vi "Read Done_.vi"(8 "error in (no error)":errorcluster, 11 "TCPReceiver in":refnum<class "TCPReceiver.lvclass">) -> (0 "error out":errorcluster, 2 "Done?":bool, 3 "TCPReceiver out":refnum<class "TCPReceiver.lvclass">)   [LabVIEW 2019, in "TCPReceiver.lvclass"]
uses:
  TCPReceiver.lvclass
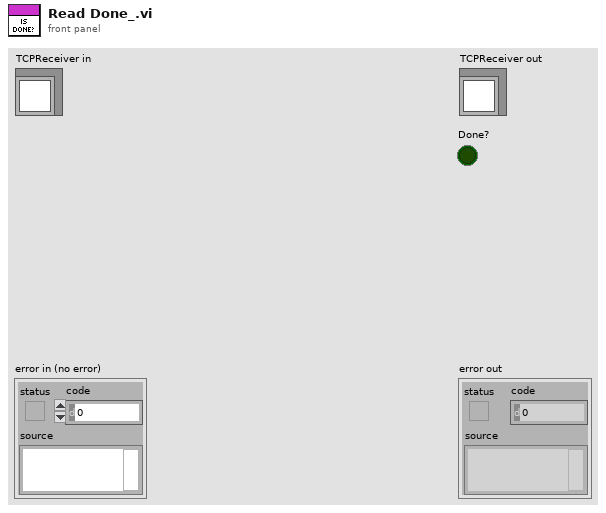
[diagram p1: front panel]
types:
  T1 = typedef "TCPReceiver.lvclass/TCPReceiver Progress STYP.ctl" = cluster{"HeaderSize?":bool, "Header?":bool, "Body?":bool}
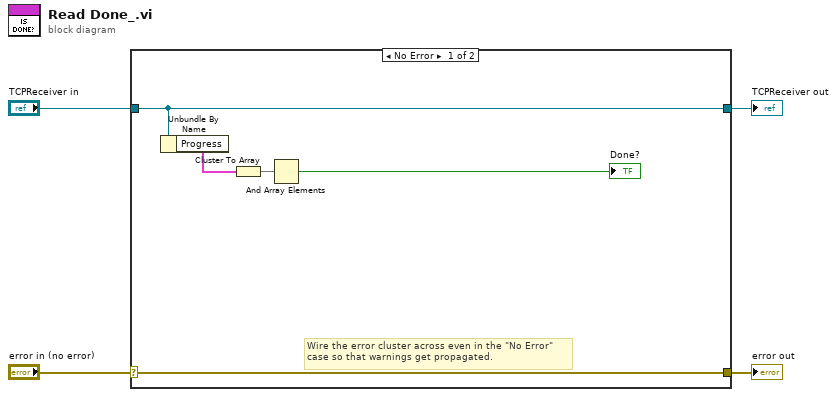
[diagram p0: block diagram]
diagram:
  n1 = case shown="No Error" "error in (no error)" {
    selector: "error in (no error)" -> [w9 w11]
    tunnel: [w9 w11] -> w3
    tunnel: [w8 w10] -> w1
    tunnel: "TCPReceiver in" -> [w8 w10]
    frame No Error {
      # "Wire the error cluster across even in the \"No Error\"\ncase so that warnings get propagated."
      n2 = Unbundle By Name(w8) -> ("Progress"=w7:T1)
      n3 = Cluster To Array(cluster=w7) -> (array=w6:bool[])
      n4 = And Array Elements(Boolean array=w6) -> (logical AND=→"Done?":bool)
    }
    frame Error {
    }
  }
  "error out" <- w3
  "TCPReceiver out" <- w1
